vi "To Network Byte Order U32.vi"(7 "network byte order":u32) -> (3 "native byte order":u32)   [LabVIEW 2020, in "NI_WFCN.lvlib"]
doc: "Convert U32 IPv4 address from network byte order to native byte order."
uses:
  <vilib>/net/WFCN/NI_WFCN.lvlib
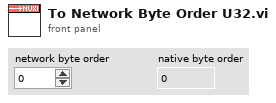
[diagram p1: front panel]
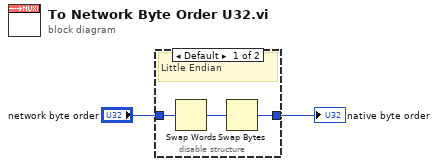
[diagram p0: block diagram]
diagram:
  n1 = disable-structure shown="Default" {
    disable-tunnel: "network byte order" -> [w5 w6]
    disable-tunnel: [w4 w6] -> w2
    frame condition #0 (active) {
      # "Little Endian"
      n2 = Swap Words(1:w5) -> (0:w3:u32)
      n3 = Swap Bytes(anything=w3) -> (byte swapped=w4:u32)
    }
    frame condition #1 {
      # "Big Endian"
    }
  }
  "native byte order" <- w2
